vi "testFlattenAccelerationToXML.vi"() -> ()   [LabVIEW 2016, in "UnitsAndXML.lvlib"]
uses:
  <userlib>/Common/UnitsAndXML/UnitsAndXML.lvlib
  <userlib>/Common/UnitsAndXML/FlattenItemWithUnitToXML/FlattenAccelerationToXML/AccelerationUnit.ctl
  <userlib>/Common/UnitsAndXML/FlattenItemWithUnitToXML/FlattenAccelerationToXML/typeMethods/flattenAccelerationToXML_Array.vi
  <userlib>/Common/UnitsAndXML/FlattenItemWithUnitToXML/FlattenAccelerationToXML/typeMethods/flattenAccelerationToXML_Scalar.vi
panel:
  out "error out":errorcluster
  in  "accelerationUnitInXML":T1
  out "xmlStringArray":string
  out "xmlStringScalar":string
  in  "acceleration":dbl[unit][](array[numeric])=[14.999999999999998, 29.999999999999996, 45.0, 59.99999999999999]
  in  "acceleration":dbl[unit]=14.999999999999998
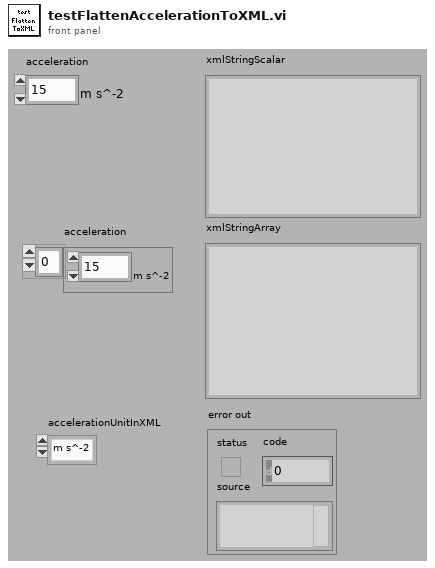
[diagram p1: front panel]
types:
  T1 = typedef "UnitsAndXML.lvlib/AccelerationUnit.ctl" = enum16{"m s^-2"}
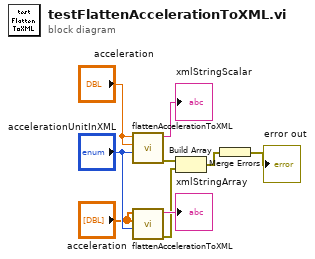
[diagram p0: block diagram]
diagram:
  n1 = call-poly <userlib>:"flattenAccelerationToXML.vi"("accelerationUnitInXML"="accelerationUnitInXML", "accelerationAgain"="acceleration", "acceleration"="acceleration") -> ("error out"=w6:errorcluster, "xmlString"=→"xmlStringScalar":string)  [unwired: 7 in]
  n2 = call-poly <userlib>:"flattenAccelerationToXML.vi"("accelerationUnitInXML"="accelerationUnitInXML", 10:"acceleration"="acceleration", 11:"acceleration"="acceleration") -> ("error out"=w1:errorcluster, "xmlString"=→"xmlStringArray":string)  [unwired: 7 in]
  n3 = Build Array(w6, w1) -> (w7:errorcluster[])
  n4 = Merge Errors(w7) -> (→"error out":errorcluster)
